vi "sv_Level View (1 Ch).vi"(4 "reference resistance [Ohm]":dbl=600.0, 6 "carrier level [EU^2 rms]":dbl=1.0, 7 "desired units":T7(ring)=enum."EU rms", 8 "error in (no error)":errorcluster, 9 "spectrum info":T1={"channel name"="", "description"="", "x-axis units"=0, "spectral info"={"spectrum type"=enum."Power [Magnitude^2]", "linear/dB"=enum."linear", "window"=0, "window size"=0, "FFT size"=0}, "engineering units"=0, "custom label"="", "dB reference [EU]"=0.0, "peak units"=enum."rms", "weighting filter"=0, "spectral density?"=FALSE, "unit label"="", "spectrum skewed?"=FALSE, "complimentary spectrum units"=enum."none"} {"x-axis units" items=["Time (s)"=0, "Frequency-CB (Hz)"=1, "Frequency-CPB (Hz)"=1248, "Frequency-Arbitrary (Hz)"=2357, "Quefrency (s)"=2, "Revolutions (rev)"=3, "Order"=4, "Speed (RPM)"=11, "Speed (rad/s)"=21, "Index"=65535]; "weighting filter" items=["Linear", "A-weighting", "B-weighting", "C-weighting", "ITU-R 468-4", "Dolby", "CCITT", "C-message", "Wb", "Wc", "Wd", "We", "Wf", "Wh", "Wj", "Wk", "Wm", "AES17 20 kHz lowpass", "AES17 40 kHz lowpass", "AES17 20 kHz highpass", "AES17 40 kHz highpass"]; "dB reference [EU]" format="%.2f"; "engineering units" items=["custom..."=0, "V"=1, "A"=21, "C"=30, "pC"=31, "s"=32, "-"=29, "Pa"=2, "N"=20, "g"=3, "m/s^2"=4, "m/s"=5, "m"=6, "mm/s"=12, "mm"=13, "micron/s"=14, "micron"=15, "in/s^2"=7, "in/s"=8, "in"=9, "mil/s"=10, "mil"=11, "rad/s^2"=16, "rad/s"=17, "rad"=18, "deg/s^2"=26, "deg/s"=27, "deg"=28, "RPM"=22, "cycle/s^2"=23, "Hz"=24, "cycle"=25, "strain"=19]; "spectral info"."window" items=["None "=0, "Hanning"=1, "Hamming"=2, "Blackman-Harris"=3, "Exact Blackman"=4, "Blackman"=5, "Flat Top"=6, "4 Term B-Harris "=7, "7 Term B-Harris"=8, "Low Sidelobe"=9, "Force - Exponential"=10, "Gaussian"=62]}, 11 "level [EU^2 rms]":dbl format="%_5f") -> (0 "error out":errorcluster, 3 "converted level":dbl format="%_4f", 5 "unit label":string)   [LabVIEW 2017, in "SoundVib_Distortion.lvlib"]
doc: "Use this VI to convert power level to desired units.\n\nNote: All conversions to dB use power formula 10*log(P/Pref) because input level should be in power units (EU^2 rms)."
uses:
  <vilib>/addons/Sound and Vibration/svt_Distortion/SoundVib_Distortion.lvlib
  <vilib>/addons/_NISVFA/_Shared subVIs/Controls/svc_Spectrum Info.ctl
  <vilib>/addons/_NISVFA/_Shared subVIs/Controls/svc_X-Axis Units.ctl
  <vilib>/addons/_NISVFA/_Shared subVIs/Controls/svc_Spectrum Type.ctl
  <vilib>/addons/_NISVFA/_Shared subVIs/Controls/svc_Engineering Units Text Ring.ctl
  <vilib>/addons/_NISVFA/_Shared subVIs/Controls/svc_Weighting Filter Text Ring.ctl
  <vilib>/addons/_NISVFA/_Shared subVIs/Controls/svc_Complimentary Spectrum Units.ctl
  <vilib>/addons/_NISVFA/_Shared subVIs/Common/svc_Get Weighting Enum and Labels.vi
  <vilib>/addons/_NISVFA/_Shared subVIs/Common/svc_Unit Label Lexical Class.vi
  <vilib>/addons/_NISVFA/_Shared subVIs/Common/svc_Engineering Units to Unit Label.vi
  <vilib>/addons/_NISVFA/_Shared subVIs/Common/svc_Format Value (DBL).vi
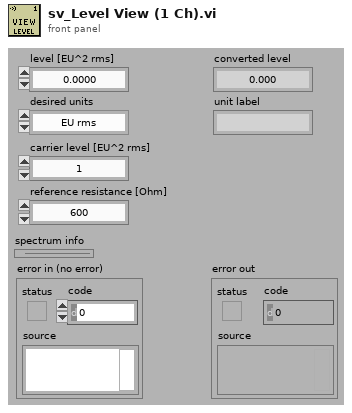
[diagram p1: front panel]
types:
  T1 = typedef "svc_Spectrum Info.ctl" = cluster{"channel name":string, "description":string, "x-axis units":T2, "spectral info":cluster{"spectrum type":T3, "linear/dB":enum16{"linear", "dB"}, "window":u16, "window size":i32, "FFT size":i32}, "engineering units":T4, "custom label":string, "dB reference [EU]":dbl, "peak units":enum16{"rms", "peak", "peak-peak"}, "weighting filter":T5, "spectral density?":bool, "unit label":string, "spectrum skewed?":bool, "complimentary spectrum units":T6}
  T2 = typedef "svc_X-Axis Units.ctl" = u16
  T3 = typedef "svc_Spectrum Type.ctl" = enum16{"FFT Spectrum [complex]", "Amplitude [Magnitude]", "Power [Magnitude^2]", "Cross Spectrum [complex]", "Frequency Response [Complex]"}
  T4 = typedef "svc_Engineering Units Text Ring.ctl" = u16
  T5 = typedef "svc_Weighting Filter Text Ring.ctl" = u16
  T6 = typedef "svc_Complimentary Spectrum Units.ctl" = enum16{"none", "radians", "degrees", "cycles", "imaginary"}
  T7 = enum16{"EU^2 rms", "EU rms", "dB", "dBc", "dBV", "dBu", "dBm"}
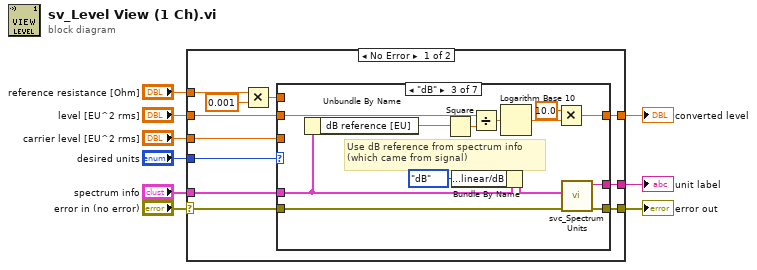
[diagram p0: block diagram]
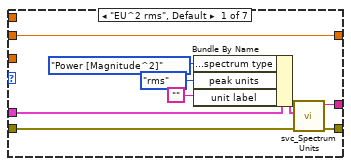
[diagram p2: hidden frame]
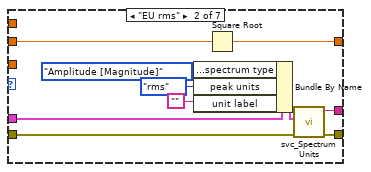
[diagram p3: hidden frame]
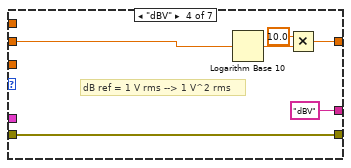
[diagram p4: hidden frame]
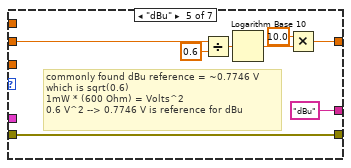
[diagram p5: hidden frame]
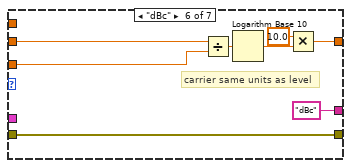
[diagram p6: hidden frame]
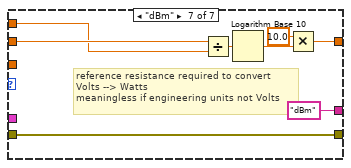
[diagram p7: hidden frame]
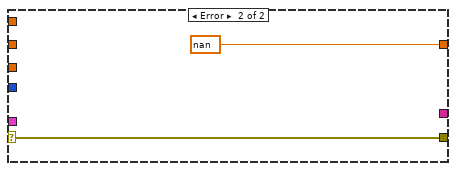
[diagram p8: hidden frame]
diagram:
  n1 = case shown="No Error" "error in (no error)" {
    selector: "error in (no error)" -> [w12 w83]
    tunnel: [w11 _] -> w9
    tunnel: [w20 nan ("peak amplitude [EU pk]")] -> w8
    tunnel: "level [EU^2 rms]" -> [w19 _]
    tunnel: "desired units" -> [w18 _]
    tunnel: [w10 w83] -> w4
    tunnel: "spectrum info" -> [w13 _]
    tunnel: "carrier level [EU^2 rms]" -> [w17 _]
    tunnel: "reference resistance [Ohm]" -> [w16 _]
    frame No Error {
      n2 = Multiply(x=w16, y=0.001) -> (x*y=w14:dbl)
      n3 = case shown="\"dB\"" w18 {
        tunnel: w19 -> [w29 w39 w52 w55 w66 w74 w82]
        tunnel: [w29 w38 w47 w56 w62 w70 w78] -> w20
        tunnel: w17 -> [_ _ _ _ _ w69 _]
        tunnel: w14 -> [_ _ _ _ _ _ w77]
        tunnel: w13 -> [w27 w33 w41 _ _ _ _]
        tunnel: w12 -> [w25 w37 w46 w53 w60 w68 w76]
        tunnel: [w24 w35 w44 "dBV" ("unit label") "dBu" ("unit label") "dBc" ("unit label") "dBm" ("unit label")] -> w11
        tunnel: [w23 w36 w45 w53 w60 w68 w76] -> w10
        frame "EU^2 rms", Default {
          n4 = Bundle By Name(cluster=w27, "spectral info.spectrum type"=svc_Spectrum_Type."Power [Magnitude^2]", "peak units"=enum16{"rms", "peak", "peak-peak"}."rms", "unit label"="") -> (w26:T1)
          n5 = call <vilib>:"svc_Spectrum Units.vi"("error in (no error)"=w25, "spectrum info in"=w26) -> ("error out"=w23:errorcluster, "unit label"=w24:string)  [unwired: 2 in, 2 out]
        }
        frame "EU rms" {
          n6 = Bundle By Name(cluster=w33, "spectral info.spectrum type"=svc_Spectrum_Type."Amplitude [Magnitude]", "peak units"=enum16{"rms", "peak", "peak-peak"}."rms", "unit label"="") -> (w32:T1)
          n7 = Square Root(x=w39) -> (sqrt(x)=w38:dbl)
          n8 = call <vilib>:"svc_Spectrum Units.vi"("error in (no error)"=w37, "spectrum info in"=w32) -> ("error out"=w36:errorcluster, "unit label"=w35:string)  [unwired: 2 in, 2 out]
        }
        frame "dB" {
          # "Use dB reference from spectrum info \n(which came from signal)"
          n9 = Unbundle By Name(w41) -> ("dB reference [EU]"=w43:dbl)
          n10 = Square(x=w43) -> (x^2=w51:dbl)
          n11 = Bundle By Name(cluster=w41, "spectral info.linear/dB"=enum16{"linear", "dB"}."dB") -> (w40:T1)
          n12 = Divide(x=w52, y=w51) -> (x/y=w50:dbl)
          n13 = Logarithm Base 10(1:w50) -> (0:w49:dbl)
          n14 = Multiply(x=10.0 ("y"), y=w49) -> (x*y=w47:dbl)
          n15 = call <vilib>:"svc_Spectrum Units.vi"("error in (no error)"=w46, "spectrum info in"=w40) -> ("error out"=w45:errorcluster, "unit label"=w44:string)  [unwired: 2 in, 2 out]
        }
        frame "dBV" {
          # "dB ref = 1 V rms --> 1 V^2 rms"
          n16 = Logarithm Base 10(1:w55) -> (0:w58:dbl)
          n17 = Multiply(x=10.0 ("y"), y=w58) -> (x*y=w56:dbl)
        }
        frame "dBu" {
          # "commonly found dBu reference = ~0.7746 V\nwhich is sqrt(0.6)\n1mW * (600 Ohm) = Volts^2\n0.6 V^2 --> 0.7746 V is reference for dBu"
          n18 = Divide(x=w66, y=0.6) -> (x/y=w65:dbl)
          n19 = Logarithm Base 10(1:w65) -> (0:w64:dbl)
          n20 = Multiply(x=10.0 ("y"), y=w64) -> (x*y=w62:dbl)
        }
        frame "dBc" {
          # "carrier same units as level"
          n21 = Divide(x=w74, y=w69) -> (x/y=w73:dbl)
          n22 = Logarithm Base 10(1:w73) -> (0:w72:dbl)
          n23 = Multiply(x=10.0 ("y"), y=w72) -> (x*y=w70:dbl)
        }
        frame "dBm" {
          # "reference resistance required to convert \nVolts --> Watts\nmeaningless if engineering units not Volts"
          n24 = Divide(x=w82, y=w77) -> (x/y=w81:dbl)
          n25 = Logarithm Base 10(1:w81) -> (0:w80:dbl)
          n26 = Multiply(x=10.0 ("y"), y=w80) -> (x*y=w78:dbl)
        }
      }
    }
    frame Error {
    }
  }
  "unit label" <- w9
  "converted level" <- w8
  "error out" <- w4
